vi "ke37xx Configure Measurement Buffer.vi"(0 "VISA Resource Name":refnum<visa-resource-name>, 5 "Buffer Name":string, 7 "Collect Channels (True)":bool=TRUE, 9 "Collect Time Stamps (True)":bool=TRUE, 11 "error in (no error)":errorcluster) -> (4 "VISA Resource Name Out":refnum<visa-resource-name>, 15 "error out":errorcluster)   [LabVIEW 2009, in "Keithley 3700 Series.lvlib"]
doc: "This VI allows you to configure various aspects of an existing measurement buffer."
uses:
  <instrlib>/Keithley 3706/Keithley 3700 Series.lvlib
panel:
  in  "Append Mode (False)":bool
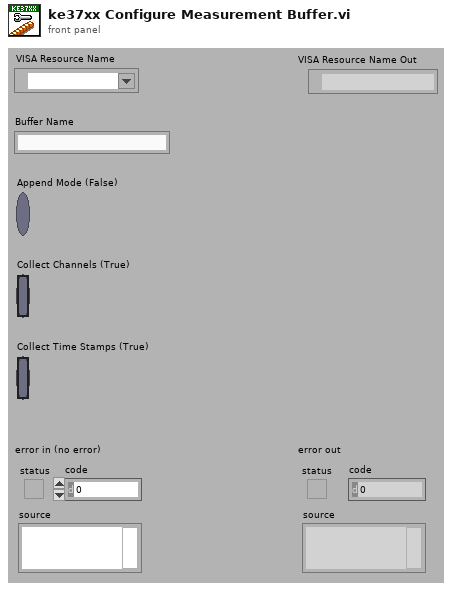
[diagram p1: front panel]
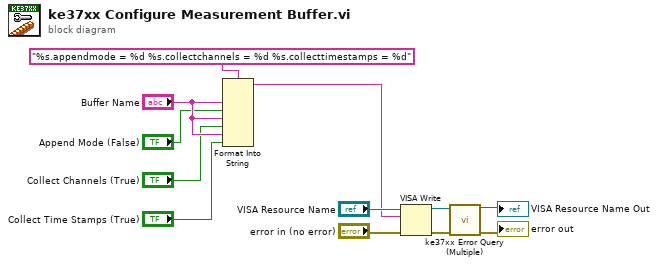
[diagram p0: block diagram]
diagram:
  n1 = Format Into String(format string="%s.appendmode = %d %s.collectchannels = %d %s.collecttimestamps = %d", "Buffer Name", "Append Mode (False)", "Buffer Name", "Collect Channels (True)", "Buffer Name", "Collect Time Stamps (True)") -> (resulting string=w5:string)  [unwired: 2 in, 1 out]
  n2 = VISA Write(VISA resource name="VISA Resource Name", write buffer=w5, error in (no error)="error in (no error)") -> (VISA resource name out=w10:refnum<visa-resource-name>, error out=w8:errorcluster)  [unwired: 1 out]
  n3 = call <instrlib>:"ke37xx Error Query (Multiple).vi"("VISA resource name"=w10, "error in (no error)"=w8) -> ("VISA resource name out"=→"VISA Resource Name Out":refnum<visa-resource-name>, "error out"=→"error out":errorcluster)  [unwired: 12 out]
